vi "获取PID参数.vi"(7 "字符串":string) -> (0 "PID":sgl[](array[numeric]))   [LabVIEW 2016]
panel:
  out "实际值":u32
  out "实际值字符串":string
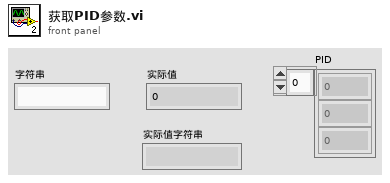
[diagram p1: front panel]
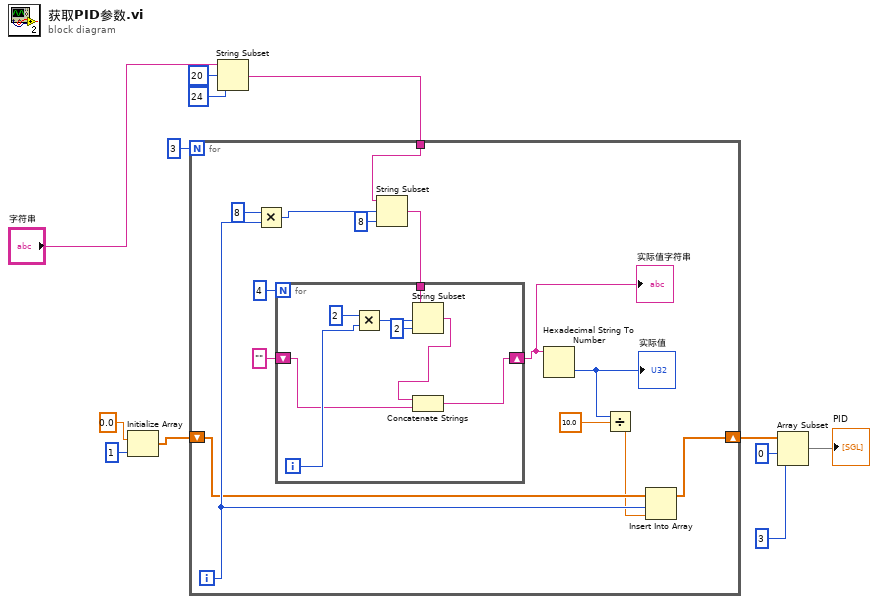
[diagram p0: block diagram]
diagram:
  n1 = Initialize Array(sgl 0.0, 1 ("维数大小")) -> (w5:sgl[])
  n2 = String Subset(string="字符串", offset (0)=20 ("偏移量(0)"), length (rest)=24 ("长度（剩余）")) -> (substring=w9:string)
  n3 = for {
    N: 3 -> [_]
    tunnel: w9 -> [w23]
    shift-right: [w16] -> w4
    shift-left: w5 -> [w17]
    i -> [w18]
    n4 = Multiply(x=8, y=w18) -> (x*y=w21:i32)
    n5 = String Subset(string=w23, offset (0)=w21, length (rest)=8 ("长度（剩余）")) -> (substring=w19:string)
    n6 = for {
      N: 4 -> [_]
      shift-right: [w34] -> w24
      shift-left: "" -> [w27]
      tunnel: w19 -> [w33]
      i -> [w32]
      n7 = Multiply(x=2, y=w32) -> (x*y=w30:i32)
      n8 = String Subset(string=w33, offset (0)=w30, length (rest)=2 ("长度（剩余）")) -> (substring=w28:string)
      n9 = Concatenate Strings(w28, w27) -> (w34:string)
    }
    "实际值字符串" <- w24
    n10 = Hexadecimal String To Number(string=w24) -> (number=w15:u32)  [unwired: 2 in, 1 out]
    "实际值" <- w15
    n11 = Divide(x=w15, y=sgl 10.0) -> (x/y=w13:sgl)
    n12 = Insert Into Array(array=w17, index=w18, new element=w13) -> (w16:sgl[])
  }
  n13 = Array Subset(array=w4, index=0 ("索引"), length=3 ("长度")) -> (→"PID":sgl[])
